vi "AFG Wait for Complete.vi"(8 "error in (no error)":errorcluster, 10 "Delay":u32, 11 "Actor_AFG in":refnum<class "Actor_AFG.lvclass">) -> (0 "error out":errorcluster, 3 "Actor_AFG out":refnum<class "Actor_AFG.lvclass">)   [LabVIEW 2020, in "Actor_AFG.lvlib" / "Actor_AFG.lvclass"]
uses:
  Actor_AFG.lvclass
  C:/Program Files/National Instruments/LabVIEW 2020/vi.lib/ActorFramework/Actor/Actor.lvclass
  AFG_Event.ctl
  Actor_AFG.lvclass/Actor_AFG.ctl
  <vilib>/ActorFramework/Actor/Actor.lvclass/Actor.ctl
  <vilib>/ActorFramework/Actor/Actor.lvclass
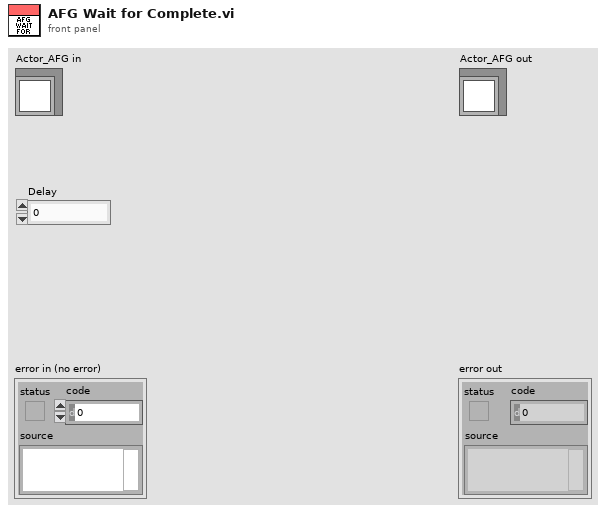
[diagram p1: front panel]
types:
  T1 = typedef "Actor_AFG.lvlib/Actor_AFG.lvclass/AFG_Event.ctl" = enum16{"General Event", "Inited", "Output", "Waveform Set", "DC Configured", "Cycle End", "Error"}
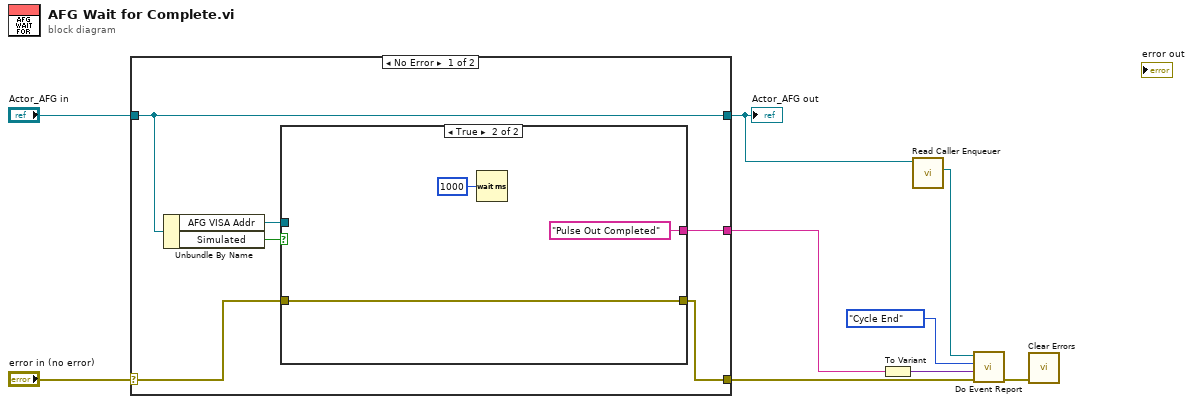
[diagram p0: block diagram]
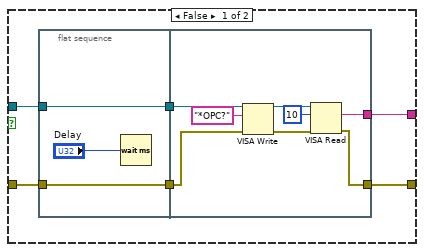
[diagram p2: hidden frame]
diagram:
  n1 = case shown="No Error" "error in (no error)" {
    selector: "error in (no error)" -> [w12 w37]
    tunnel: [w11 w37] -> w3
    tunnel: [w15 w36] -> w1
    tunnel: "Actor_AFG in" -> [w15 w36]
    tunnel: [w10 _] -> w2
    frame No Error {
      n2 = Unbundle By Name(w15) -> ("AFG VISA Addr"=w13:refnum<visa-resource-name>, "Simulated"=w14:bool)
      n3 = case shown="True" w14 {
        tunnel: w13 -> [w20 _]
        tunnel: w12 -> [w18 w35]
        tunnel: [w17 w35] -> w11
        tunnel: [w16 "Pulse Out Completed" ("read buffer")] -> w10
        frame False {
          n4 = flat-sequence {
            tunnel: [w23] -> w21
            tunnel: w20 -> [w23]
            tunnel: [w22] -> w19
            tunnel: w18 -> [w22]
            tunnel: w21 -> [w32]
            tunnel: w19 -> [w31]
            tunnel: [w27] -> w17
            tunnel: [w25] -> w16
            frame #0 {
              n5 = Wait (ms)(milliseconds to wait="Delay") -> ()  [unwired: 1 out]
            }
            frame #1 {
              n6 = VISA Write(VISA resource name=w32, write buffer="*OPC?", error in (no error)=w31) -> (VISA resource name out=w29:refnum<visa-resource-name>, error out=w28:errorcluster)  [unwired: 1 out]
              n7 = VISA Read(VISA resource name=w29, byte count=u32 10, error in (no error)=w28) -> (read buffer=w25:string, error out=w27:errorcluster)  [unwired: 2 out]
            }
          }
        }
        frame True {
          n8 = Wait (ms)(milliseconds to wait=u32 1000) -> ()  [unwired: 1 out]
        }
      }
    }
    frame Error {
    }
  }
  "Actor_AFG out" <- w1
  n9 = To Variant(anything=w2) -> (Variant=w7:variant)
  n10 = call <vilib>:"Read Caller Enqueuer.vi"("Actor"=w1) -> ("Caller Enqueuer"=w5:refnum<class "Message Enqueuer.lvclass">)  [unwired: 10 in]
  n11 = call "Do Event Report.vi"("error in (no error)"=w3, "Event Data"=w7, "Report Events"=AFG_Event."Cycle End", "Caller Enqueuer"=w5) -> ("error out"=w4:errorcluster)  [unwired: 6 in, 1 out]
  n12 = call <vilib>:"Clear Errors.vi"("error in (no error)"=w4) -> ()  [unwired: 5 in, 2 out]
